vi "Close.vi"(8 "error in (no error)":errorcluster, 11 "SGDV_Ctrl_Class in":refnum<class "SGDV_Ctrl_Class.lvclass">) -> (0 "error out":errorcluster, 3 "SGDV_Ctrl_Class out":refnum<class "SGDV_Ctrl_Class.lvclass">)   [LabVIEW 2013, in "SGDV_Ctrl_v13_lib.lvlib" / "SGDV_Ctrl_Class.lvclass"]
uses:
  SGDV_Ctrl_Class.lvclass
panel:
  # "This VI is used to turn off the power of servo drive and set the velocity to zero."
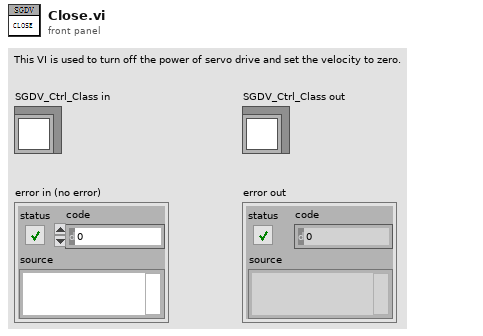
[diagram p1: front panel]
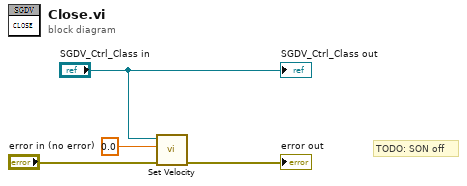
[diagram p0: block diagram]
diagram:
  # "TODO: SON off"
  n1 = call "Set Velocity.vi"("error in (no error)"="error in (no error)", "Velocity In(deg/s)"=0.0, "SGDV_Ctrl_Class in"="SGDV_Ctrl_Class in") -> ("error out"=→"error out":errorcluster)  [unwired: 7 in, 1 out]
  "SGDV_Ctrl_Class out" <- "SGDV_Ctrl_Class in"
